vi "20220114 sub 1 ABC catch select-1.vi"(0 "ABC":i32) -> (2 "ABC path out go catch":cluster{"X":dbl, "Y":dbl}[](array[cluster]))   [LabVIEW 2019]
uses:
  subVI/move/move array.ctl
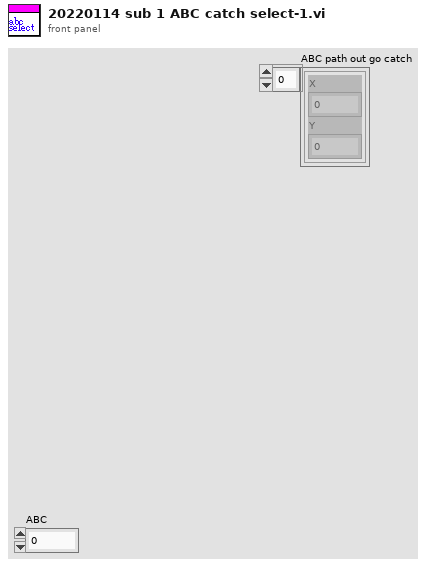
[diagram p1: front panel]
types:
  T1 = typedef "move array.ctl" = cluster{"X":dbl, "Y":dbl}[]
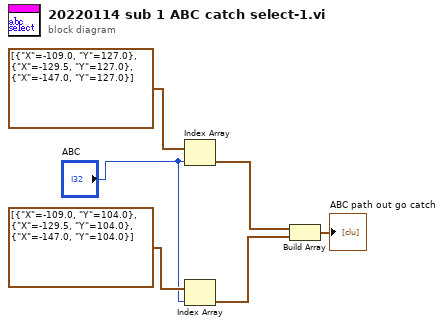
[diagram p0: block diagram]
diagram:
  n1 = Index Array(array=T1 [{"X"=-109.0, "Y"=127.0}, {"X"=-129.5, "Y"=127.0}, {"X"=-147.0, "Y"=127.0}] ("Array"), index="ABC") -> (element=w3:cluster{"X":dbl, "Y":dbl})
  n2 = Index Array(array=T1 [{"X"=-109.0, "Y"=104.0}, {"X"=-129.5, "Y"=104.0}, {"X"=-147.0, "Y"=104.0}] ("Array"), index="ABC") -> (element=w2:cluster{"X":dbl, "Y":dbl})
  n3 = Build Array(w3, w2) -> (→"ABC path out go catch":cluster{"X":dbl, "Y":dbl}[])
